vi "Autotuning wizard.vi"(6 "New PID Parameters input":T1 {"Rate (min)" format="%.4f"; "Reset (min)" format="%.4f"; "PB (%)" format="%.4f"}, 7 "tuning completed?":bool, 8 "Control":T4 {"output" format="%.2f"; "setpoint" format="%.2f"; "process variable" format="%.2f"}, 9 "options":T3={"sp low"=0.0, "sp high"=100.0, "out low"=-100.0, "out high"=100.0, "hold (F)"=FALSE, "auto (T)"=TRUE, "pro. band (F)"=FALSE, "reverse acting (T)"=TRUE, "beta"=1.0, "linearity"=1.0, "dt (s)"=-1.0} {"dt (s)" format="%.2f"; "linearity" min=0.0 max=1.0 format="%.2f"; "sp low" format="%.2f"; "sp high" format="%.2f"; "out low" format="%.2f"; "out high" format="%.2f"; "beta" min=0.0 max=1.0 format="%.2f"}, 10 "autotuning parameters":T2={"Controller Type"=0, "# of cycles to avg"=3, "Relay amplitude"=0.0, "Control design  "=0, "Noise level"=0.25} {"Noise level" format="%.2f"; "Control design" items=["Normal", "Fast", "Slow"]; "Relay amplitude" format="%.2f"; "Controller Type" items=["PID", "PI", "P"]}, 11 "current state":string) -> (0 "New PID Parameters out":T1 {"Rate (min)" format="%.4f"; "Reset (min)" format="%.4f"; "PB (%)" format="%.4f"}, 1 "complete?":bool, 2 "autotuning parameters out":T2={"Controller Type"=0, "# of cycles to avg"=3, "Relay amplitude"=0.0, "Control design  "=0, "Noise level"=0.25} {"Noise level" format="%.2f"; "Control design" items=["Normal", "Fast", "Slow"]; "Relay amplitude" format="%.2f"; "Controller Type" items=["PID", "PI", "P"]}, 3 "state":string, 4 "yes/no out":bool)   [LabVIEW 2017, in "NI_PID__autopid compat.lvlib"]
doc: "This VI serves as the user interface for the autotuning procedure."
uses:
  <vilib>/addons/control/pid/NI_PID__autopid compat.lvlib
  <vilib>/addons/control/pid/_autopid compat.llb/State.gbl.vi
panel:
  in  "help":bool
  out "yes/no":bool
  in  "Accept":bool
  in  "Re-estimate":bool
  in  "current parameters":T5={"Controller Type"=0, "# of cycles to avg"=3, "Relay amplitude"=0.0, "Control design  "=0, "Noise level %"=0.25} {"Noise level %" format="%.2f"; "Control design" items=["Normal", "Fast", "Slow"]; "Relay amplitude" format="%.2f"; "Controller Type" items=["PID", "PI", "P"]}
  in  "cancel":bool
  in  "next":bool
  in  "back":bool
  in  "states":T6(ring)=enum."Start"
  out "VI name":string
  in  "Current noise level estimate":dbl format="%.2f"
  out "New PID Parameters":T7 {"Td (min)" format="%.4f"; "Ti (min)" format="%.4f"; "Kc (or PB%)" format="%.4f"}
  in  "OK":bool
  out "Control chart":T8(graph)
  out "Dialog":string
  in  "no":bool
  in  "yes":bool
  # "PID Autotuning Wizard"
  # "SP & PV range:"
  # "Output range:"
  # "-1: default,using\nsystem clock"
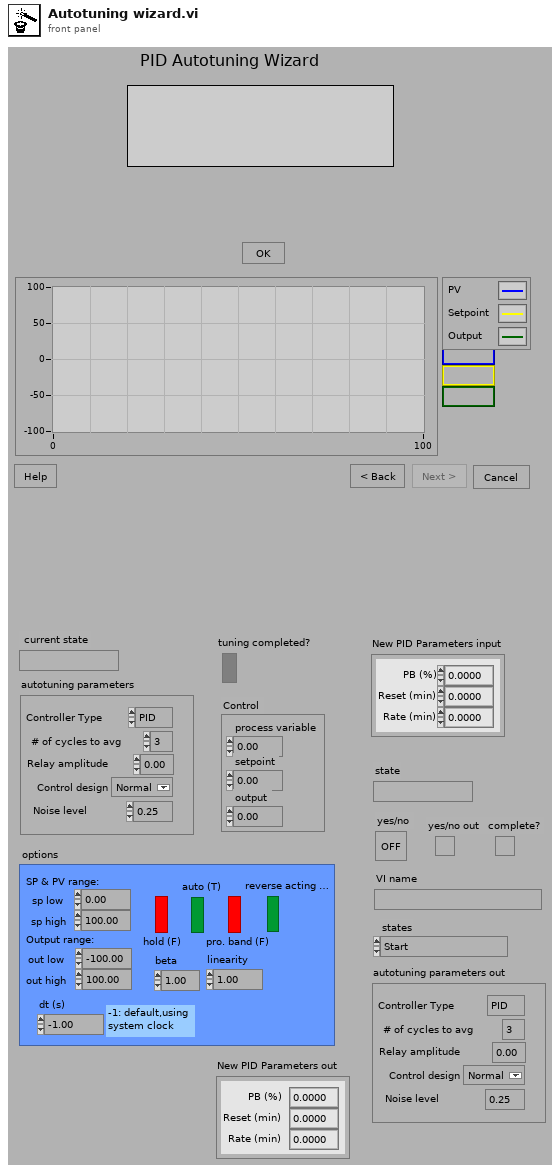
[diagram p1: front panel]
types:
  T1 = cluster{"PB (%)":dbl, "Reset (min)":dbl, "Rate (min)":dbl, "Index":i32}
  T2 = cluster{"Controller Type":u16, "# of cycles to avg":i32, "Relay amplitude":dbl, "Control design  ":u16, "Noise level":dbl}
  T3 = cluster{"sp low":dbl, "sp high":dbl, "out low":dbl, "out high":dbl, "hold (F)":bool, "auto (T)":bool, "pro. band (F)":bool, "reverse acting (T)":bool, "beta":dbl, "linearity":dbl, "dt (s)":dbl}
  T4 = cluster{"process variable":dbl, "setpoint":dbl, "output":dbl}
  T5 = cluster{"Controller Type":u16, "# of cycles to avg":i32, "Relay amplitude":dbl, "Control design  ":u16, "Noise level %":dbl}
  T6 = enum16{"Normal", "Start", "Check params", "Check noise", "Start noise est.", "Re-estimate noise", "Begin autotune", "Autotuning", "New parameters", ""}
  T7 = cluster{"Kc (or PB%)":dbl, "Ti (min)":dbl, "Td (min)":dbl, "Index":i32}
  T8 = cluster{"PV%":dbl, "setpoint (%)":dbl, "output (%)":dbl}
  T9 = cluster{"PV%":dbl, "setpoint (%)":dbl, "output (%)":dbl}[]
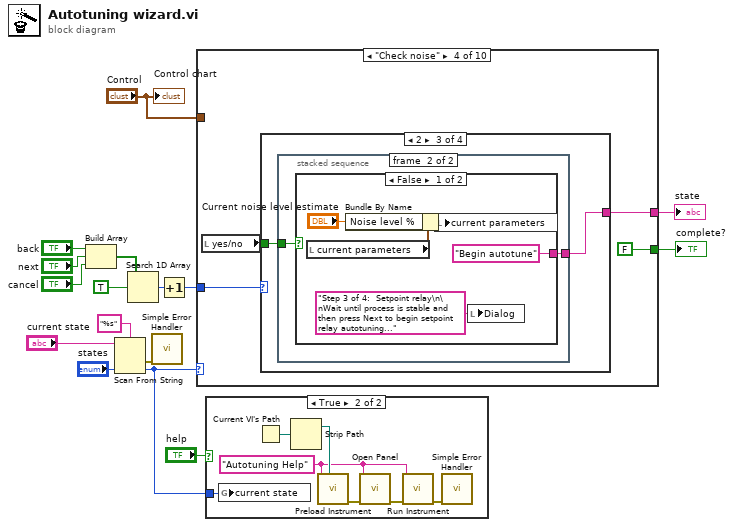
[diagram p0: block diagram]
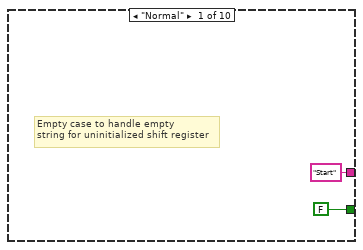
[diagram p3: hidden frame]
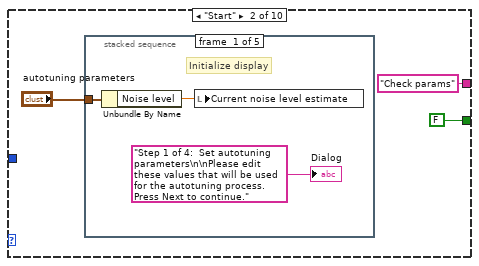
[diagram p4: hidden frame]
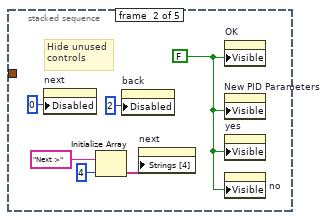
[diagram p5: hidden frame]
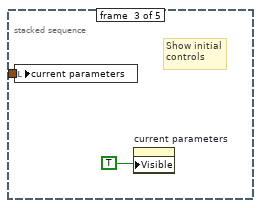
[diagram p6: hidden frame]
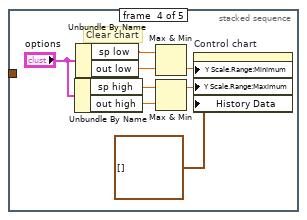
[diagram p7: hidden frame]
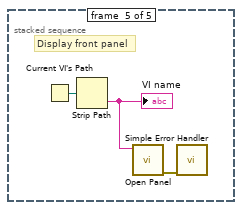
[diagram p8: hidden frame]
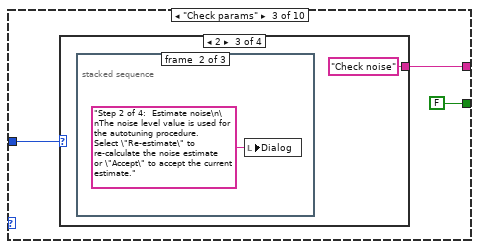
[diagram p9: hidden frame]
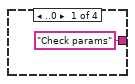
[diagram p10: hidden frame]
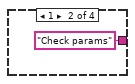
[diagram p11: hidden frame]
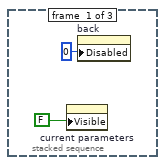
[diagram p12: hidden frame]
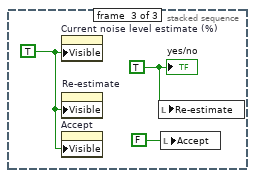
[diagram p13: hidden frame]
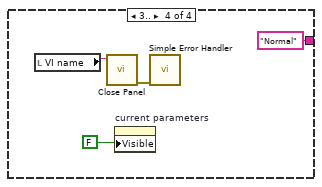
[diagram p14: hidden frame]
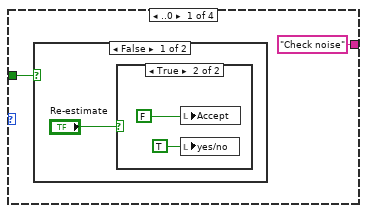
[diagram p15: hidden frame]
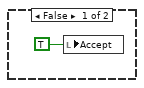
[diagram p16: hidden frame]
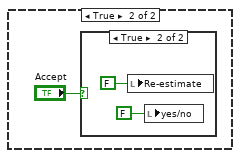
[diagram p17: hidden frame]
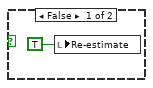
[diagram p18: hidden frame]
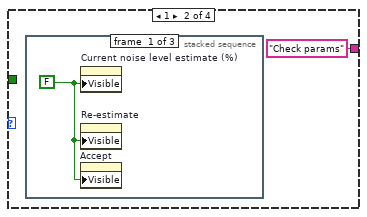
[diagram p19: hidden frame]
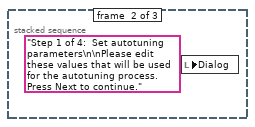
[diagram p20: hidden frame]
diagram:
  n1 = Build Array("back", "next", "cancel") -> (w13:bool[])
  n2 = Scan From String(format string="%s", input string="current state", default 1="states") -> (error out=w16:errorcluster, output 1=w1:T6)  [unwired: 2 in, 2 out]
  n3 = Search 1D Array(1D array=w13, element=TRUE) -> (index of element=w12:i32)  [unwired: 1 out]
  n4 = call <vilib>:"Simple Error Handler.vi"("error in (no error)"=w16) -> ()  [unwired: 1 in, 8 out]
  n5 = Increment(x=w12) -> (x+1=w7:i32)
  n6 = case shown="\"Check noise\"" w1 {
    tunnel: ["Start" "Check params" w44 w61 w95 w110 w129 w147 w183 "Start"] -> w5
    tunnel: [FALSE FALSE FALSE FALSE FALSE FALSE FALSE FALSE w182 FALSE] -> w3
    tunnel: w7 -> [_ _ w45 w62 w96 w111 w130 w148 w184 _]
    tunnel: "Control" -> [_ _ _ _ _ w109 _ _ _ _]
    frame "Normal" {
      # "Empty case to handle empty\nstring for uninitialized shift register"
    }
    frame "Start" {
      n7 = stacked-sequence {
        tunnel: "autotuning parameters" -> [w24 _ w31 _ _]
        frame #0 {
          # "Initialize display"
          n8 = Unbundle By Name(w24) -> ("Noise level"=w23:dbl)
          n9 = local write "Current noise level estimate"(w23) -> ()
          "Dialog" <- "Step 1 of 4:  Set autotuning parameters\n\nPlease edit these values that will be used for the autotuning process.  Press Next to continue." ("Dialog")
        }
        frame #1 {
          w30 = FALSE ("Visible")
          # "Hide unused\ncontrols"
          n10 = property on="next" class="Bool"("Disabled"=u8 0) -> ()  [unwired: 2 in, 2 out]
          n11 = Initialize Array("Next >", 4) -> (w25:string[])
          n12 = property on="back" class="Bool"("Disabled"=u8 2) -> ()  [unwired: 2 in, 2 out]
          n13 = property on="next" class="Bool"("Strings [4]"=w25) -> ()  [unwired: 2 in, 2 out]
          n14 = property on="OK" class="Bool (strict)"("Visible"=w30) -> ()  [unwired: 2 in, 2 out]
          n15 = property on="New PID Parameters" class="Clust (strict)"("Visible"=w30) -> ()  [unwired: 2 in, 2 out]
          n16 = property on="yes" class="Bool (strict)"("Visible"=w30) -> ()  [unwired: 2 in, 2 out]
          n17 = property on="no" class="Bool (strict)"("Visible"=w30) -> ()  [unwired: 2 in, 2 out]
        }
        frame #2 {
          # "Show initial\ncontrols"
          n18 = local write "current parameters"(w31) -> ()
          n19 = property on="current parameters" class="Clust (strict)"("Visible"=TRUE) -> ()  [unwired: 2 in, 2 out]
        }
        frame #3 {
          # "Clear chart"
          n20 = Unbundle By Name("options") -> ("sp high"=w38:dbl, "out high"=w37:dbl)
          n21 = Unbundle By Name("options") -> ("sp low"=w39:dbl, "out low"=w40:dbl)
          n22 = Max & Min(x=w39, y=w40) -> (min(x,y)=w36:dbl)  [unwired: 1 out]
          n23 = Max & Min(x=w38, y=w37) -> (max(x,y)=w35:dbl)  [unwired: 1 out]
          n24 = property on="Control chart" class="WFChart (strict)"("Y Scale.Range:Minimum"=w36, "Y Scale.Range:Maximum"=w35, "History Data"=T9 []) -> ()  [unwired: 2 in, 2 out]
        }
        frame #4 {
          # "Display front panel"
          n25 = Current VI's Path() -> (path=w42:path)
          n26 = Strip Path(path=w42) -> (name=w41:string)  [unwired: 1 out]
          "VI name" <- w41
          n27 = call <vilib>:"Open Panel.vi"("VI name"=w41) -> ("error out"=w43:errorcluster)  [unwired: 2 in, 8 out]
          n28 = call <vilib>:"Simple Error Handler.vi"("error in (no error)"=w43) -> ()  [unwired: 1 in, 8 out]
        }
      }
    }
    frame "Check params" {
      n29 = case shown="2" w45 {
        tunnel: ["Check params" "Check params" "Check noise" "Normal"] -> w44
        frame ..0 {
        }
        frame 1 {
        }
        frame 2 {
          n30 = stacked-sequence {
            frame #0 {
              n31 = property on="current parameters" class="Clust (strict)"("Visible"=FALSE) -> ()  [unwired: 2 in, 2 out]
              n32 = property on="back" class="Bool"("Disabled"=u8 0) -> ()  [unwired: 2 in, 2 out]
            }
            frame #1 {
              n33 = local write "Dialog"("Step 2 of 4:  Estimate noise\n\nThe noise level value is used for the autotuning procedure.  Select \"Re-estimate\" to re-calculate the noise estimate or \"Accept\" to accept the current estimate." ("Dialog")) -> ()
            }
            frame #2 {
              w54 = TRUE ("yes/no")
              w55 = TRUE ("Visible")
              n34 = property on="Current noise level estimate (%)" class="DigNum (strict)"("Visible"=w55) -> ()  [unwired: 2 in, 2 out]
              n35 = property on="Re-estimate" class="Bool (strict)"("Visible"=w55) -> ()  [unwired: 2 in, 2 out]
              n36 = property on="Accept" class="Bool (strict)"("Visible"=w55) -> ()  [unwired: 2 in, 2 out]
              n37 = local write "Re-estimate"(w54) -> ()
              n38 = local write "Accept"(FALSE ("Accept")) -> ()
              "yes/no" <- w54
            }
          }
        }
        frame 3.. {
          n39 = local read "VI name"() -> (w57:string)
          n40 = call <vilib>:"Close Panel.vi"("VI name"=w57) -> ("error out"=w58:errorcluster)  [unwired: 1 in, 9 out]
          n41 = property on="current parameters" class="Clust (strict)"("Visible"=FALSE) -> ()  [unwired: 2 in, 2 out]
          n42 = call <vilib>:"Simple Error Handler.vi"("error in (no error)"=w58) -> ()  [unwired: 1 in, 8 out]
        }
      }
    }
    frame "Check noise" {
      n43 = local read "yes/no"() -> (w60:bool)
      n44 = case shown="2" w62 {
        tunnel: ["Check noise" "Check params" w79 "Normal"] -> w61
        tunnel: w60 -> [w64 _ w80 _]
        frame ..0 {
          n45 = case shown="False" w64 {
            frame False {
              n46 = case shown="True" "Re-estimate" {
                frame False {
                  n47 = local write "Accept"(TRUE ("Accept")) -> ()
                }
                frame True {
                  n48 = local write "Accept"(FALSE ("Re-estimate")) -> ()
                  n49 = local write "yes/no"(TRUE ("yes/no")) -> ()
                }
              }
            }
            frame True {
              n50 = case shown="True" "Accept" {
                frame False {
                  n51 = local write "Re-estimate"(TRUE ("Re-estimate")) -> ()
                }
                frame True {
                  n52 = local write "Re-estimate"(FALSE ("Re-estimate")) -> ()
                  n53 = local write "yes/no"(FALSE ("yes/no")) -> ()
                }
              }
            }
          }
        }
        frame 1 {
          n54 = stacked-sequence {
            frame #0 {
              w75 = FALSE ("Visible")
              n55 = property on="Current noise level estimate (%)" class="DigNum (strict)"("Visible"=w75) -> ()  [unwired: 2 in, 2 out]
              n56 = property on="Re-estimate" class="Bool (strict)"("Visible"=w75) -> ()  [unwired: 2 in, 2 out]
              n57 = property on="Accept" class="Bool (strict)"("Visible"=w75) -> ()  [unwired: 2 in, 2 out]
            }
            frame #1 {
              n58 = local write "Dialog"("Step 1 of 4:  Set autotuning parameters\n\nPlease edit these values that will be used for the autotuning process.  Press Next to continue." ("Dialog")) -> ()
            }
            frame #2 {
              n59 = property on="current parameters" class="Clust (strict)"("Visible"=TRUE) -> ()  [unwired: 2 in, 2 out]
              n60 = property on="back" class="Bool"("Disabled"=u8 2) -> ()  [unwired: 2 in, 2 out]
            }
          }
        }
        frame 2 {
          n61 = stacked-sequence {
            tunnel: w80 -> [_ w83]
            tunnel: [_ w82] -> w79
            frame #0 {
              w81 = FALSE ("Visible")
              n62 = property on="Current noise level estimate (%)" class="DigNum (strict)"("Visible"=w81) -> ()  [unwired: 2 in, 2 out]
              n63 = property on="Re-estimate" class="Bool (strict)"("Visible"=w81) -> ()  [unwired: 2 in, 2 out]
              n64 = property on="Accept" class="Bool (strict)"("Visible"=w81) -> ()  [unwired: 2 in, 2 out]
            }
            frame #1 {
              n65 = case shown="False" w83 {
                tunnel: ["Begin autotune" "Start noise est."] -> w82
                frame False {
                  n66 = local read "current parameters"() -> (w84:T5)
                  n67 = Bundle By Name(cluster=w84, "Noise level %"="Current noise level estimate") -> (w86:T5)
                  n68 = local write "current parameters"(w86) -> ()
                  n69 = local write "Dialog"("Step 3 of 4:  Setpoint relay\n\nWait until process is stable and then press Next to begin setpoint relay autotuning..." ("Dialog")) -> ()
                }
                frame True {
                  n70 = local write "Dialog"("Step 2 of 4:  Estimate noise\n\nMake sure process variable is stabilized, then press Next" ("Dialog")) -> ()
                }
              }
            }
          }
        }
        frame 3.. {
          w91 = FALSE ("Visible")
          n71 = property on="Current noise level estimate (%)" class="DigNum (strict)"("Visible"=w91) -> ()  [unwired: 2 in, 2 out]
          n72 = property on="Re-estimate" class="Bool (strict)"("Visible"=w91) -> ()  [unwired: 2 in, 2 out]
          n73 = property on="Accept" class="Bool (strict)"("Visible"=w91) -> ()  [unwired: 2 in, 2 out]
          n74 = local read "VI name"() -> (w93:string)
          n75 = call <vilib>:"Close Panel.vi"("VI name"=w93) -> ("error out"=w94:errorcluster)  [unwired: 1 in, 9 out]
          n76 = call <vilib>:"Simple Error Handler.vi"("error in (no error)"=w94) -> ()  [unwired: 1 in, 8 out]
        }
      }
    }
    frame "Start noise est." {
      n77 = case shown="1" w96 {
        tunnel: ["Start noise est." "Check noise" "Re-estimate noise" "Normal"] -> w95
        frame ..0 {
        }
        frame 1 {
          n78 = stacked-sequence {
            frame #0 {
              w100 = TRUE ("Visible")
              n79 = property on="Current noise level estimate (%)" class="DigNum (strict)"("Visible"=w100) -> ()  [unwired: 2 in, 2 out]
              n80 = property on="Re-estimate" class="Bool (strict)"("Visible"=w100) -> ()  [unwired: 2 in, 2 out]
              n81 = property on="Accept" class="Bool (strict)"("Visible"=w100) -> ()  [unwired: 2 in, 2 out]
            }
            frame #1 {
              n82 = local write "Dialog"("Step 2 of 4:  Estimate noise\n\nThe noise level value is used for the autotuning procedure.  Select \"Re-estimate\" to re-calculate the noise estimate or \"Accept\" to accept the current estimate." ("Dialog")) -> ()
            }
          }
        }
        frame 2 {
          n83 = call <vilib>:"MeaNoise.vi"("OK"=FALSE) -> ()  [unwired: 1 in, 2 out]
          n84 = local write "Dialog"("Step 2 of 4:  Estimate noise\n\nWait at least ten cycles, then press Next again." ("Dialog")) -> ()
        }
        frame 3.. {
          n85 = local read "VI name"() -> (w106:string)
          n86 = call <vilib>:"Close Panel.vi"("VI name"=w106) -> ("error out"=w107:errorcluster)  [unwired: 1 in, 9 out]
          n87 = call <vilib>:"Simple Error Handler.vi"("error in (no error)"=w107) -> ()  [unwired: 1 in, 8 out]
        }
      }
    }
    frame "Re-estimate noise" {
      n88 = Unbundle By Name(w109) -> ("process variable"=w108:dbl)
      n89 = case shown="2" w111 {
        tunnel: ["Re-estimate noise" "Start noise est." "Check noise" "Normal"] -> w110
        tunnel: w108 -> [w113 _ _ _]
        frame ..0 {
          n90 = call <vilib>:"MeaNoise.vi"("OK"=TRUE, "PV %"=w113) -> ()  [unwired: 2 out]
        }
        frame 1 {
          n91 = local write "Dialog"("Step 2 of 4:  Estimate noise\n\nMake sure process variable is stabilized, then press Next" ("Dialog")) -> ()
        }
        frame 2 {
          n92 = stacked-sequence {
            frame #0 {
              n93 = call <vilib>:"MeaNoise.vi"("OK"=FALSE) -> ("Noise"=w119:dbl)  [unwired: 1 in, 1 out]
              n94 = local write "Current noise level estimate"(w119) -> ()
            }
            frame #1 {
              w122 = FALSE ("yes/no")
              w123 = TRUE ("Visible")
              n95 = property on="Current noise level estimate (%)" class="DigNum (strict)"("Visible"=w123) -> ()  [unwired: 2 in, 2 out]
              n96 = property on="Re-estimate" class="Bool (strict)"("Visible"=w123) -> ()  [unwired: 2 in, 2 out]
              n97 = property on="Accept" class="Bool (strict)"("Visible"=w123) -> ()  [unwired: 2 in, 2 out]
              n98 = local write "Re-estimate"(w122) -> ()
              n99 = local write "yes/no"(w122) -> ()
              n100 = local write "Accept"(TRUE ("Accept")) -> ()
            }
            frame #2 {
              n101 = local write "Dialog"("Step 2 of 4:  Estimate noise\n\nThe noise level value is used for the autotuning procedure.  Select \"Re-estimate\" to re-calculate the noise estimate or \"Accept\" to accept the current estimate." ("Dialog")) -> ()
            }
          }
        }
        frame 3.. {
          n102 = local read "VI name"() -> (w126:string)
          n103 = call <vilib>:"Close Panel.vi"("VI name"=w126) -> ("error out"=w127:errorcluster)  [unwired: 1 in, 9 out]
          n104 = call <vilib>:"Simple Error Handler.vi"("error in (no error)"=w127) -> ()  [unwired: 1 in, 8 out]
        }
      }
    }
    frame "Begin autotune" {
      n105 = case shown="1" w130 {
        tunnel: ["Begin autotune" "Check noise" "Autotuning" "Normal"] -> w129
        frame ..0 {
        }
        frame 1 {
          n106 = stacked-sequence {
            frame #0 {
              w134 = TRUE ("Visible")
              n107 = property on="Current noise level estimate (%)" class="DigNum (strict)"("Visible"=w134) -> ()  [unwired: 2 in, 2 out]
              n108 = property on="Re-estimate" class="Bool (strict)"("Visible"=w134) -> ()  [unwired: 2 in, 2 out]
              n109 = property on="Accept" class="Bool (strict)"("Visible"=w134) -> ()  [unwired: 2 in, 2 out]
            }
            frame #1 {
              n110 = local write "Dialog"("Step 2 of 4:  Estimate noise\n\nThe noise level value is used for the autotuning procedure.  Select \"Re-estimate\" to re-calculate the noise estimate or \"Accept\" to accept the current estimate." ("Dialog")) -> ()
            }
          }
        }
        frame 2 {
          n111 = property on="OK" class="Bool (strict)"("Visible"=TRUE, "Disabled"=u8 0) -> ()  [unwired: 2 in, 2 out]
          n112 = local write "OK"(FALSE ("OK")) -> ()
          n113 = local write "Dialog"("Step 3 of 4:  Setpoint relay\n\nSetpoint relay in progress... Press OK when process variable oscillations are steady." ("Dialog")) -> ()
          n114 = property on="next" class="Bool"("Disabled"=u8 2) -> ()  [unwired: 2 in, 2 out]
        }
        frame 3.. {
          n115 = local read "VI name"() -> (w143:string)
          n116 = call <vilib>:"Close Panel.vi"("VI name"=w143) -> ("error out"=w144:errorcluster)  [unwired: 1 in, 9 out]
          n117 = call <vilib>:"Simple Error Handler.vi"("error in (no error)"=w144) -> ()  [unwired: 1 in, 8 out]
        }
      }
      n118 = local read "current parameters"() -> (→"autotuning parameters out":T5)
    }
    frame "Autotuning" {
      n119 = case shown="..0" w148 {
        tunnel: [w158 "Check noise" "Autotuning" "Normal"] -> w147
        frame ..0 {
          n120 = case shown="True" "tuning completed?" {
            tunnel: ["Autotuning" w160] -> w158
            frame False {
            }
            frame True {
              n121 = stacked-sequence {
                tunnel: [_ _ "New parameters" _] -> w160
                frame #0 {
                  n122 = local write "yes/no"(TRUE ("yes/no")) -> ()
                  n123 = local write "OK"(FALSE ("OK")) -> ()
                  n124 = property on="OK" class="Bool (strict)"("Visible"=FALSE, "Disabled"=u8 0) -> ()  [unwired: 2 in, 2 out]
                  "New PID Parameters" <- "New PID Parameters input"
                }
                frame #1 {
                  w166 = TRUE ("Visible")
                  n125 = property on="New PID Parameters" class="Clust (strict)"("Visible"=w166) -> ()  [unwired: 2 in, 2 out]
                  n126 = property on="yes" class="Bool (strict)"("Visible"=w166) -> ()  [unwired: 2 in, 2 out]
                  n127 = property on="no" class="Bool (strict)"("Visible"=w166) -> ()  [unwired: 2 in, 2 out]
                }
                frame #2 {
                  n128 = local write "Dialog"("Step 4 of 4:  New PID gains\n\nNew PID parameters have been calculated.  You may accept or reject the values." ("Dialog")) -> ()
                }
                frame #3 {
                  n129 = property on="next" class="Bool"("Disabled"=u8 0) -> ()  [unwired: 2 in, 2 out]
                  n130 = Initialize Array("Exit", 4) -> (w170:string[])
                  n131 = property on="next" class="Bool"("Strings [4]"=w170) -> ()  [unwired: 2 in, 2 out]
                }
              }
            }
          }
        }
        frame 1 {
          n132 = stacked-sequence {
            frame #0 {
              w176 = TRUE ("Visible")
              n133 = property on="Current noise level estimate (%)" class="DigNum (strict)"("Visible"=w176) -> ()  [unwired: 2 in, 2 out]
              n134 = property on="Re-estimate" class="Bool (strict)"("Visible"=w176) -> ()  [unwired: 2 in, 2 out]
              n135 = property on="Accept" class="Bool (strict)"("Visible"=w176) -> ()  [unwired: 2 in, 2 out]
              n136 = property on="next" class="Bool"("Disabled"=u8 0) -> ()  [unwired: 2 in, 2 out]
              n137 = property on="OK" class="Bool (strict)"("Visible"=FALSE) -> ()  [unwired: 2 in, 2 out]
            }
            frame #1 {
              n138 = local write "Dialog"("Step 2 of 4:  Estimate noise\n\nThe noise level value is used for the autotuning procedure.  Select \"Re-estimate\" to re-calculate the noise estimate or \"Accept\" to accept the current estimate." ("Dialog")) -> ()
            }
          }
        }
        frame 2 {
        }
        frame 3.. {
          n139 = local read "VI name"() -> (w180:string)
          n140 = call <vilib>:"Close Panel.vi"("VI name"=w180) -> ("error out"=w181:errorcluster)  [unwired: 1 in, 9 out]
          n141 = call <vilib>:"Simple Error Handler.vi"("error in (no error)"=w181) -> ()  [unwired: 1 in, 8 out]
        }
      }
      n142 = local write "yes/no"("OK") -> ()
      n143 = case shown="True" "OK" {
        tunnel: "current parameters" -> [_ w156]
        frame False {
        }
        frame True {
          n144 = Unbundle By Name(w156) -> ("# of cycles to avg"=w155:i32)
          n145 = property on="OK" class="Bool (strict)"("Disabled"=u8 2) -> ()  [unwired: 2 in, 2 out]
          n146 = Number To Decimal String(number=w155) -> (decimal integer string=w154:string)  [unwired: 1 out]
          n147 = Concatenate Strings("Please wait (approximately " ("Dialog"), w154, " cycles)..." ("Dialog")) -> (w151:string)
          n148 = local write "Dialog"(w151) -> ()
        }
      }
      "yes/no out" <- "OK"
    }
    frame "New parameters" {
      n149 = case shown="..0" w184 {
        tunnel: ["New parameters" "Begin autotune" "Normal" "Normal"] -> w183
        tunnel: [FALSE FALSE TRUE FALSE] -> w182
        frame ..0 {
          n150 = local read "yes/no"() -> (w185:bool)
          n151 = case shown="True" w185 {
            frame False {
              n152 = case shown="True" "yes" {
                frame False {
                  n153 = local write "no"(TRUE ("Accept")) -> ()
                }
                frame True {
                  n154 = local write "yes/no"(TRUE ("yes/no")) -> ()
                  n155 = local write "no"(FALSE ("Re-estimate")) -> ()
                }
              }
            }
            frame True {
              n156 = case shown="False" "no" {
                frame False {
                  n157 = local write "yes"(TRUE ("Re-estimate")) -> ()
                }
                frame True {
                  n158 = local write "yes/no"(FALSE ("yes/no")) -> ()
                  n159 = local write "yes"(FALSE ("Re-estimate")) -> ()
                }
              }
            }
          }
        }
        frame 1 {
          n160 = stacked-sequence {
            frame #0 {
              w198 = FALSE ("Visible")
              n161 = property on="New PID Parameters" class="Clust (strict)"("Visible"=w198) -> ()  [unwired: 2 in, 2 out]
              n162 = property on="yes" class="Bool (strict)"("Visible"=w198) -> ()  [unwired: 2 in, 2 out]
              n163 = property on="no" class="Bool (strict)"("Visible"=w198) -> ()  [unwired: 2 in, 2 out]
            }
            frame #1 {
              n164 = local write "Dialog"("Step 3 of 4:  Setpoint relay\n\nWait until process is stable and then press Next to begin setpoint relay autotuning..." ("Dialog")) -> ()
            }
            frame #2 {
              n165 = Initialize Array("Next >", 4) -> (w200:string[])
              n166 = property on="next" class="Bool"("Strings [4]"=w200) -> ()  [unwired: 2 in, 2 out]
            }
          }
        }
        frame 2 {
          n167 = local read "New PID Parameters"() -> (→"New PID Parameters out":T7)
          n168 = local read "yes/no"() -> (w204:bool)
          n169 = local write "yes/no out"(w204) -> ()
          n170 = local read "VI name"() -> (w205:string)
          n171 = call <vilib>:"Close Panel.vi"("VI name"=w205) -> ("error out"=w206:errorcluster)  [unwired: 1 in, 9 out]
          n172 = call <vilib>:"Simple Error Handler.vi"("error in (no error)"=w206) -> ()  [unwired: 1 in, 8 out]
        }
        frame 3.. {
          n173 = local read "VI name"() -> (w211:string)
          n174 = call <vilib>:"Close Panel.vi"("VI name"=w211) -> ("error out"=w212:errorcluster)  [unwired: 1 in, 9 out]
          n175 = call <vilib>:"Simple Error Handler.vi"("error in (no error)"=w212) -> ()  [unwired: 1 in, 8 out]
        }
      }
    }
    frame "" {
      # "Empty case to handle empty\nstring for uninitialized shift register"
    }
  }
  "state" <- w5
  "complete?" <- w3
  n176 = case shown="True" "help" {
    tunnel: w1 -> [_ w218]
    frame False {
    }
    frame True {
      w215 = "Autotuning Help" ("VI name")
      n177 = global write "State.gbl.vi" "current state"(w218) -> ()
      n178 = Current VI's Path() -> (path=w221:path)
      n179 = Strip Path(path=w221) -> (stripped path=w220:path)  [unwired: 1 out]
      n180 = call <vilib>:"Preload Instrument.vi"("VI path"=w220, "VI name"=w215) -> ("error out"=w217:errorcluster)  [unwired: 1 in, 8 out]
      n181 = call <vilib>:"Open Panel.vi"("error in (no error)"=w217, "VI name"=w215) -> ("error out"=w216:errorcluster)  [unwired: 1 in, 8 out]
      n182 = call <vilib>:"Run Instrument.vi"("error in (no error)"=w216, "VI name"=w215) -> ("error out"=w219:errorcluster)  [unwired: 9 out]
      n183 = call <vilib>:"Simple Error Handler.vi"("error in (no error)"=w219) -> ()  [unwired: 1 in, 8 out]
    }
  }
  "Control chart" <- "Control"
